vi "QUBE ROTPEN Encoders to Angles.vi"(10 "pen enc (counts)":i32, 11 "arm enc (counts)":i32) -> (1 "alpha_full (rad)":dbl, 2 "alpha (rad)":dbl, 3 "theta (rad)":dbl)   [LabVIEW 2018]
uses:
  <vilib>/Simulation/Implementation/Shared/SIMSCR Execution Mode.ctl
  <vilib>/Simulation/Scripting/Companion Diagram/SimConfigNode/SimParams.ctl
  <vilib>/Simulation/Scripting/Companion Diagram/SimConfigNode/_simSolvers.ctl
  <vilib>/Simulation/Param Hierarchy/Typedefs/SIMPH Param Control Actions.ctl
  <vilib>/Simulation/Implementation/Shared/NILVSim_ParamChanged.vi
  <vilib>/Simulation/Implementation/Shared/NILVSIM_BeginStep.vi
  <vilib>/Simulation/SignalArithmetic/Implementation/NILVSim Gain.llb/SIM Gain (scalar).vi
  <vilib>/Simulation/Implementation/Shared/NILVSim_Manager.vi
  <vilib>/Utility/error.llb/Clear Errors.vi
  <vilib>/Simulation/Implementation/Shared/NILVSim_FinalizeModel.vi
  <vilib>/Simulation/Implementation/Shared/SIM Unbundle Sim Info.vi
  <vilib>/Simulation/Implementation/Shared/SIMSH Read Queue.vi
  <vilib>/Simulation/Implementation/Shared/NILVSim_Initialize.vi
  <vilib>/Simulation/Utility/Implementation/NILVSim Get Time and IsAcceptedStep.vi
  <vilib>/Simulation/Implementation/Shared/NILVSim_GetModelError.vi
  <vilib>/Simulation/Implementation/Shared/SIM SimErrorHandler.vi
  <vilib>/Simulation/Implementation/Shared/SIM Bundle Sim Info.vi
  <vilib>/Simulation/Scripting/Companion Diagram/SimConfigNode/SimDog.xnode
  <vilib>/Simulation/Implementation/XNodeFramework/SimXNode/SimX.xnode
  <vilib>/Simulation/Implementation/Shared/NI_SIM_Implementation.lvlib
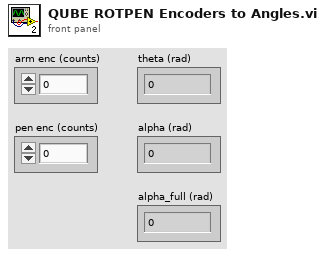
[diagram p1: front panel]
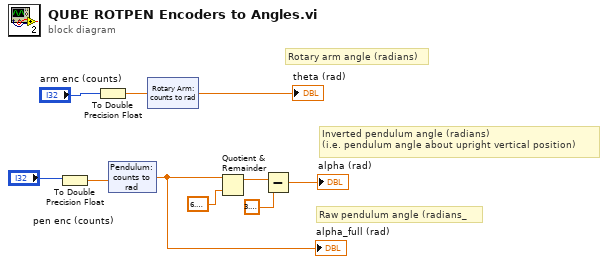
[diagram p0: block diagram]
diagram:
  # "Raw pendulum angle (radians_"
  # "Rotary arm angle (radians)"
  # "Inverted pendulum angle (radians)\n(i.e. pendulum angle about upright vertical position)"
  n1 = To Double Precision Float ("To Double Precision Float 2")(number="pen enc (counts)") -> (double precision float=w8:dbl)
  n2 = To Double Precision Float(number="arm enc (counts)") -> (double precision float=w6:dbl)
  n3 = xnode "Pendulum: \ncounts to rad"("input"=w8) -> ("output"=w9:dbl)  [unwired: 3 in]
  "alpha_full (rad)" <- w9
  n4 = xnode "Rotary Arm: \ncounts to rad"("input"=w6) -> ("output"=→"theta (rad)":dbl)  [unwired: 3 in]
  n5 = Quotient & Remainder(x=w9, y=6.283185307179586 ("Constant")) -> (x-y*floor(x/y)=w3:dbl)  [unwired: 1 out]
  n6 = Subtract(x=w3, y=3.141592653589793 ("Constant 2")) -> (x-y=→"alpha (rad)":dbl)
